vi "Initialize Bluetooth(SubVI).vi"() -> (0 "error out":errorcluster, 2 "Device Name":string, 3 "Address":string)   [LabVIEW 2014]
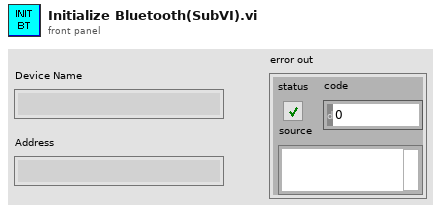
[diagram p1: front panel]
types:
  T1 = cluster{"Address":string, "Device Name":string}[]
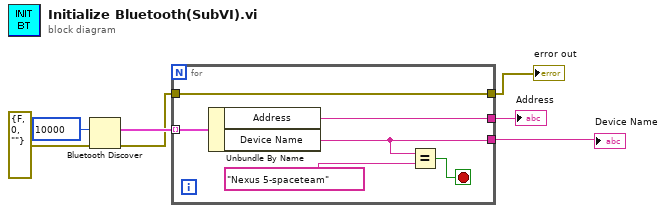
[diagram p0: block diagram]
diagram:
  n1 = Bluetooth Discover(8:errorcluster {"status"=FALSE, "code"=0, "source"=""} ("error in (no error)"), 10:10000 ("time limit ms (10000)")) -> (0:w2:errorcluster, 2:w5:T1)  [unwired: 1 out]
  n2 = for {
    tunnel: w5 -> [w13] mode=indexing
    tunnel: [w10] -> w6
    tunnel: [w9] -> w7
    tunnel: w2 -> [w8]
    tunnel: [w8] -> w1
    stop <- w11 stop-if-true
    n3 = Unbundle By Name(w13) -> ("Address"=w10:string, "Device Name"=w9:string)
    n4 = Equal?(x=w9, y="Nexus 5-spaceteam") -> (x = y?=w11:bool)
  }
  "Address" <- w6
  "Device Name" <- w7
  "error out" <- w1
